vi "Target Initialize Lookup Table Data v2.vi"(9 "error in (no error)":errorcluster) -> (1 "error out":errorcluster)   [LabVIEW 2018]
uses:
  <vilib>/Analysis/1siggen.llb/Ramp Pattern by Samples.vi
  <vilib>/Utility/file.llb/Read Delimited Spreadsheet (DBL).vi
  <vilib>/Analysis/NI_AALBase.lvlib
panel:
  out "file or folder exists?":bool
  out "All Saved Patterns \nthe same Length?":bool
  out "Theta_d":cluster{"Ramp Pattern":dbl[], "first row":dbl[]}(graph)
  out "Mean Phi":cluster{"Ramp Pattern":dbl[], "first row":dbl[]}(graph)
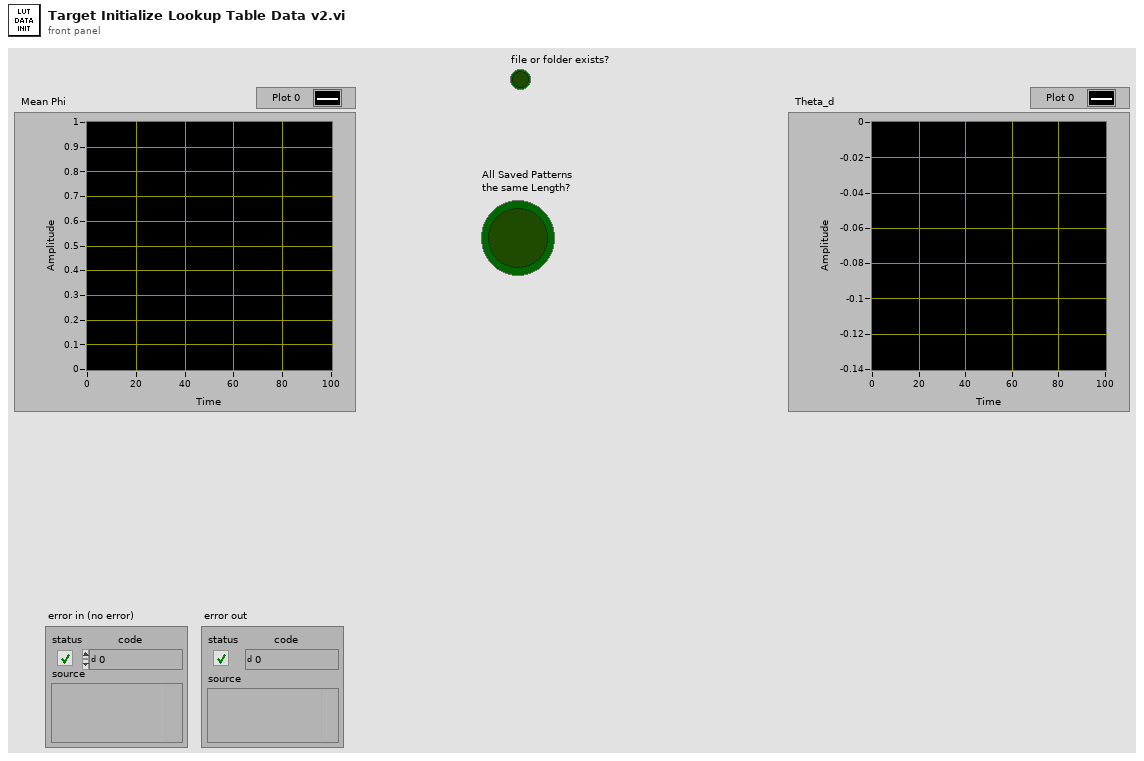
[diagram p1: front panel]
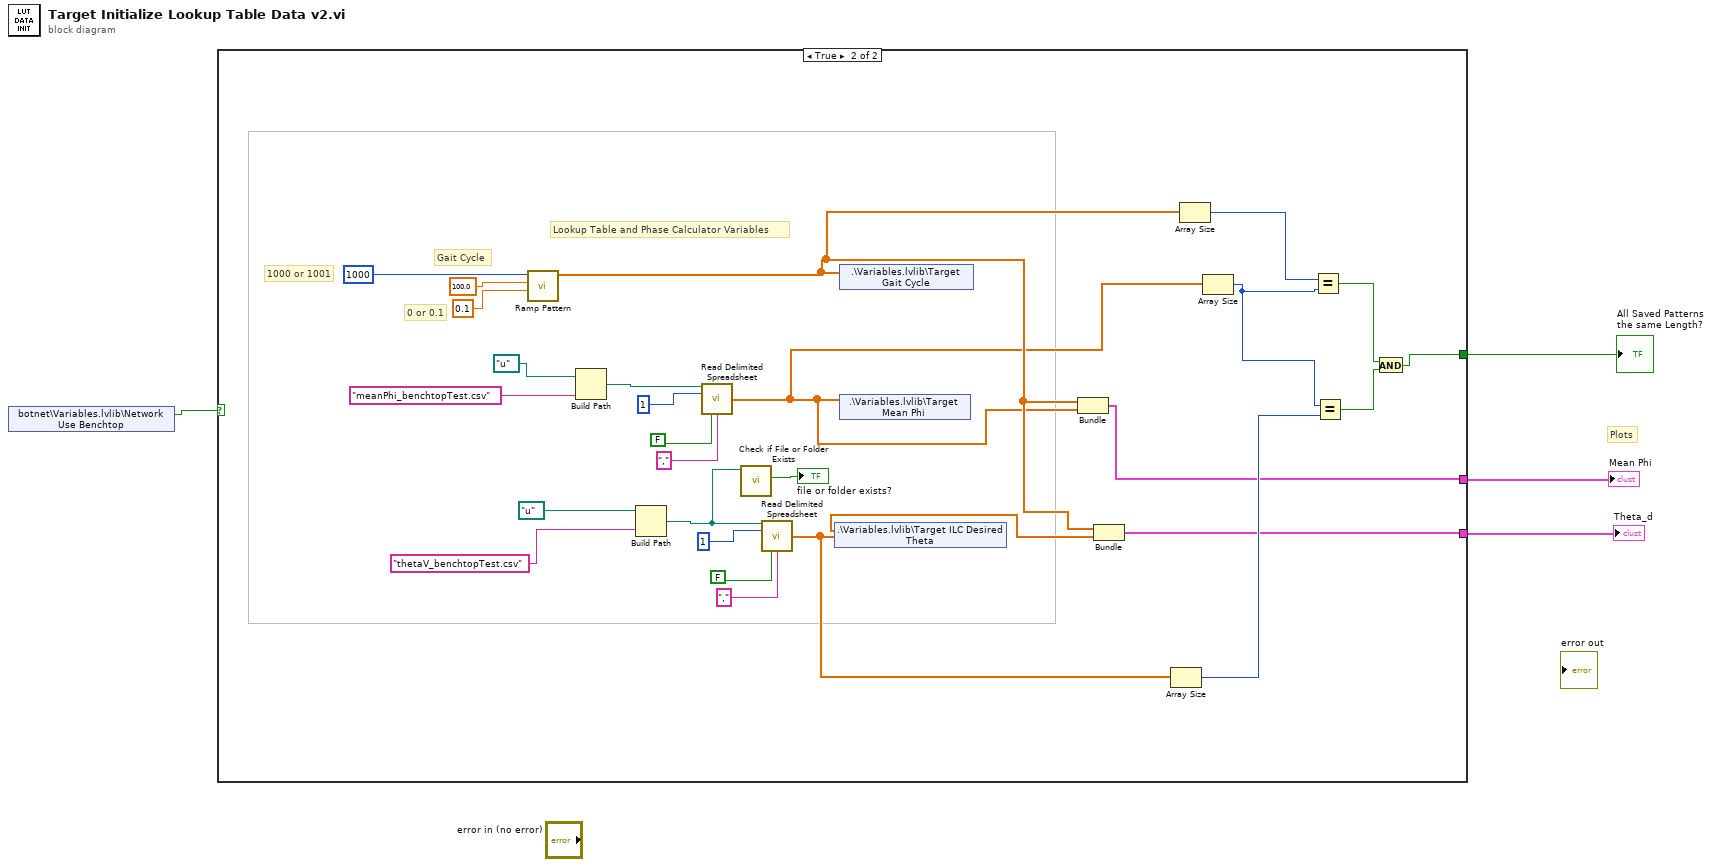
[diagram p0: block diagram]
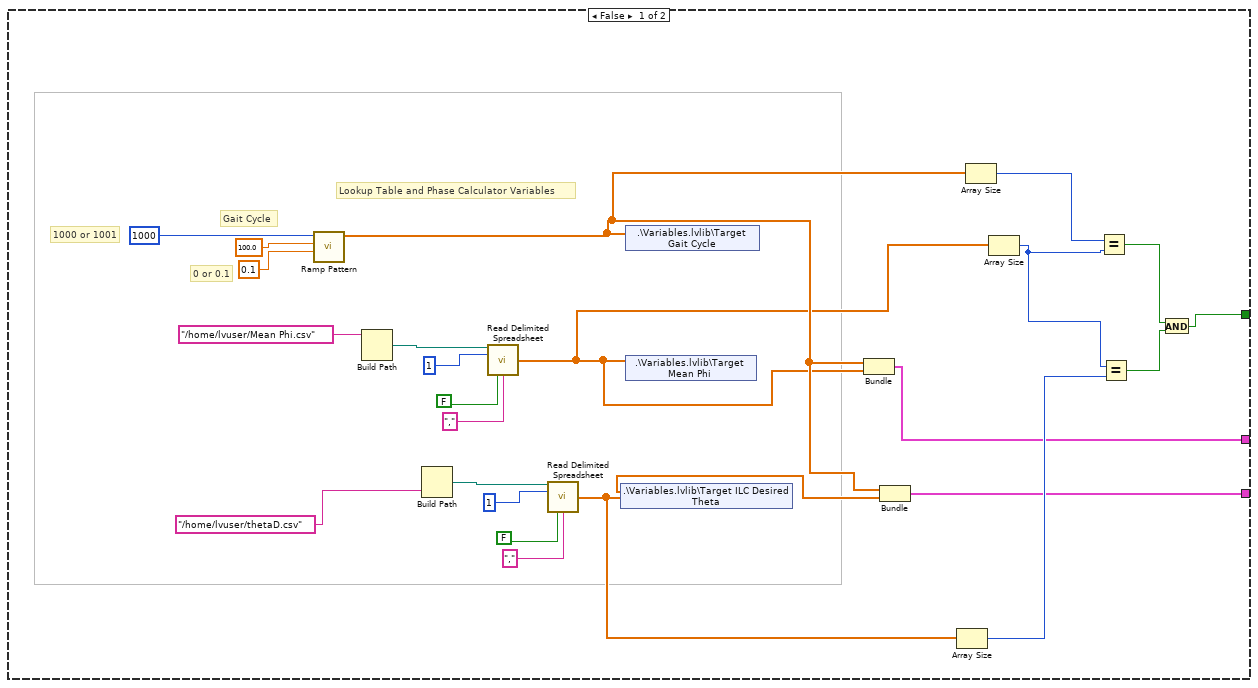
[diagram p2: hidden frame]
diagram:
  # "Plots"
  n1 = shared-variable "botnet\\Variables.lvlib\\Network Use Benchtop"() -> (w4:bool)  [unwired: 1 in, 1 out]
  n2 = case shown="True" w4 {
    tunnel: [w7 w35] -> w3
    tunnel: [w6 w33] -> w2
    tunnel: [w5 w34] -> w1
    frame False {
      # "1000 or 1001"
      # "0 or 0.1"
      # "Gait Cycle"
      # "Lookup Table and Phase Calculator Variables"
      n3 = call-poly <vilib>:"Ramp Pattern.vi"("start"=0.1, "end"=100.0, "samples"=1000) -> ("Ramp Pattern"=w15:dbl[])  [unwired: 7 in, 1 out]
      n4 = Build Path(name or relative path="/home/lvuser/Mean Phi.csv") -> (appended path=w21:path)  [unwired: 1 in]
      n5 = Build Path(name or relative path="/home/lvuser/thetaD.csv") -> (appended path=w17:path)  [unwired: 1 in]
      n6 = call-poly <vilib>:"Read Delimited Spreadsheet.vi"("file path (dialog if empty)"=w21, "number of rows (all:-1)"=1, "transpose? (F)"=FALSE, "delimiter (\\t)"="," ("delimiter (\\t)")) -> ("first row"=w14:dbl[])  [unwired: 6 in, 5 out]
      n7 = call-poly <vilib>:"Read Delimited Spreadsheet.vi"("file path (dialog if empty)"=w17, "number of rows (all:-1)"=1, "transpose? (F)"=FALSE, "delimiter (\\t)"="," ("delimiter (\\t)")) -> ("first row"=w13:dbl[])  [unwired: 6 in, 5 out]
      n8 = shared-variable ".\\Variables.lvlib\\Target ILC Desired Theta"(w13) -> ()  [unwired: 1 in, 1 out]
      n9 = shared-variable ".\\Variables.lvlib\\Target Gait Cycle"(w15) -> ()  [unwired: 1 in, 1 out]
      n10 = shared-variable ".\\Variables.lvlib\\Target Mean Phi"(w14) -> ()  [unwired: 1 in, 1 out]
      n11 = Bundle("Ramp Pattern"=w15, "first row"=w14) -> (w5:cluster{"Ramp Pattern":dbl[], "first row":dbl[]})  [unwired: 1 in]
      n12 = Bundle("Ramp Pattern"=w15, "first row"=w13) -> (w6:cluster{"Ramp Pattern":dbl[], "first row":dbl[]})  [unwired: 1 in]
      n13 = Array Size(array=w13) -> (size(s)=w10:i32)
      n14 = Array Size(array=w15) -> (size(s)=w12:i32)
      n15 = Array Size(array=w14) -> (size(s)=w11:i32)
      n16 = Equal?(x=w12, y=w11) -> (x = y?=w9:bool)
      n17 = Equal?(x=w11, y=w10) -> (x = y?=w8:bool)
      n18 = And(x=w9, y=w8) -> (x .and. y?=w7:bool)
    }
    frame True {
      # "1000 or 1001"
      # "0 or 0.1"
      # "Gait Cycle"
      # "Lookup Table and Phase Calculator Variables"
      n19 = call-poly <vilib>:"Ramp Pattern.vi"("start"=0.1, "end"=100.0, "samples"=1000) -> ("Ramp Pattern"=w43:dbl[])  [unwired: 7 in, 1 out]
      n20 = Build Path(base path=path "u:/", name or relative path="meanPhi_benchtopTest.csv") -> (appended path=w48:path)
      n21 = Build Path(base path=path "u:/", name or relative path="thetaV_benchtopTest.csv") -> (appended path=w30:path)
      n22 = call-poly <vilib>:"Read Delimited Spreadsheet.vi"("file path (dialog if empty)"=w48, "number of rows (all:-1)"=1, "transpose? (F)"=FALSE, "delimiter (\\t)"="," ("delimiter (\\t)")) -> ("first row"=w42:dbl[])  [unwired: 6 in, 5 out]
      n23 = call <vilib>:"Check if File or Folder Exists.vi"("path"=w30) -> ("file or folder exists?"=→"file or folder exists?":bool)  [unwired: 8 in, 2 out]
      n24 = call-poly <vilib>:"Read Delimited Spreadsheet.vi"("file path (dialog if empty)"=w30, "number of rows (all:-1)"=1, "transpose? (F)"=FALSE, "delimiter (\\t)"="," ("delimiter (\\t)")) -> ("first row"=w41:dbl[])  [unwired: 6 in, 5 out]
      n25 = shared-variable ".\\Variables.lvlib\\Target ILC Desired Theta"(w41) -> ()  [unwired: 1 in, 1 out]
      n26 = shared-variable ".\\Variables.lvlib\\Target Gait Cycle"(w43) -> ()  [unwired: 1 in, 1 out]
      n27 = shared-variable ".\\Variables.lvlib\\Target Mean Phi"(w42) -> ()  [unwired: 1 in, 1 out]
      n28 = Bundle("Ramp Pattern"=w43, "first row"=w42) -> (w34:cluster{"Ramp Pattern":dbl[], "first row":dbl[]})  [unwired: 1 in]
      n29 = Bundle("Ramp Pattern"=w43, "first row"=w41) -> (w33:cluster{"Ramp Pattern":dbl[], "first row":dbl[]})  [unwired: 1 in]
      n30 = Array Size(array=w41) -> (size(s)=w38:i32)
      n31 = Array Size(array=w43) -> (size(s)=w40:i32)
      n32 = Array Size(array=w42) -> (size(s)=w39:i32)
      n33 = Equal?(x=w40, y=w39) -> (x = y?=w37:bool)
      n34 = Equal?(x=w39, y=w38) -> (x = y?=w36:bool)
      n35 = And(x=w37, y=w36) -> (x .and. y?=w35:bool)
    }
  }
  "All Saved Patterns \nthe same Length?" <- w3
  "Theta_d" <- w2
  "Mean Phi" <- w1
